vi "Create Group.vi"(4 "Channel Resources (Unset)":string[](array[string]), 5 "Raw Values (F)":bool, 6 "Channel Names":string[](array[string]), 7 "Group Type":refnum<class "GroupAbstract.lvclass">, 8 "error in (no error)":errorcluster, 9 "Publish Config (None)":T1, 10 "Group Info":T2, 11 "TelemetryAPI in":refnum<class "TelemetryAPI.lvclass">) -> (0 "error out":errorcluster, 2 "Group":refnum<class "GroupAbstract.lvclass">, 3 "TelemetryAPI out":refnum<class "TelemetryAPI.lvclass">)   [LabVIEW 2020, in "Volatus.lvlib" / "TelemetryAPI.lvclass"]
uses:
  TelemetryAPI.lvclass
  lv-vecto/Vecto/Group Info.ctl
  lv-vecto/Vecto/Publish Config.ctl
  lv-vecto/Vecto/GroupAbstract/GroupAbstract.lvclass
  TelemetryAPI.lvclass/TelemetryAPI.ctl
  lv-vecto/Vecto/Channel Init.ctl
  lv-vecto/Vecto/ChannelService/Create Group Abstract.vi
  lv-vecto/Vecto/ChannelService/ChannelService.lvclass
  lv-vecto/Vecto/Group Config/Group Config.lvclass
  lv-vecto/Vecto/Vecto.lvlib
  lv-vecto/Vecto/RemoteDataService/RemoteDataService.lvclass
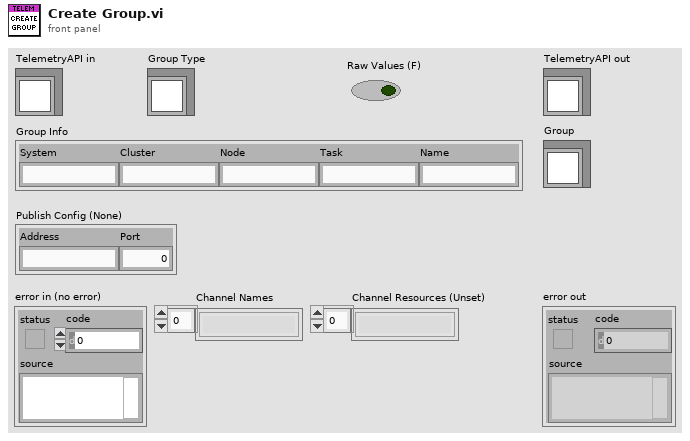
[diagram p1: front panel]
types:
  T1 = typedef "Vecto.lvlib/Publish Config.ctl" = cluster{"Address":string, "Port":u16}
  T2 = typedef "Vecto.lvlib/Group Info.ctl" = cluster{"System":string, "Cluster":string, "Node":string, "Task":string, "Name":string}
  T3 = typedef "Vecto.lvlib/Channel Init.ctl" = cluster{"Name":string, "Resource":string}
  T4 = typedef "Vecto.lvlib/Group Data Type.ctl" = enum16{"Double", "String"}
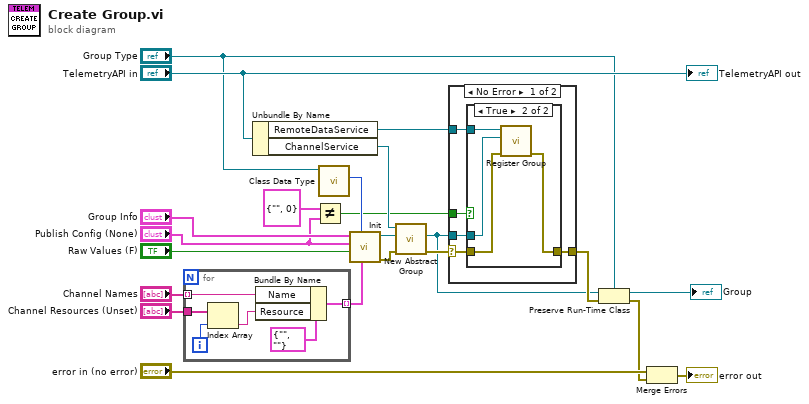
[diagram p0: block diagram]
diagram:
  n1 = for {
    tunnel: "Channel Names" -> [w24] mode=indexing
    tunnel: "Channel Resources (Unset)" -> [w27]
    tunnel: [w23] -> w13 mode=indexing
    i -> [w26]
    n2 = Index Array(array=w27, index=w26) -> (element=w25:string)
    n3 = Bundle By Name(cluster=T3 {"Name"="", "Resource"=""} ("Channel Init"), "Name"=w24, "Resource"=w25) -> (w23:T3)
  }
  n4 = Unbundle By Name("TelemetryAPI in") -> ("RemoteDataService"=w7:refnum<class "RemoteDataService.lvclass">, "ChannelService"=w19:refnum<class "ChannelService.lvclass">)
  n5 = Not Equal?(x=T1 {"Address"="", "Port"=0}, y="Publish Config (None)") -> (x != y?=w6:bool)
  n6 = call "Class Data Type.vi"("GroupAbstract in"="Group Type") -> ("Class Data Type"=w16:T4)  [unwired: 8 in, 2 out]
  n7 = call "Init.vi"("Channels"=w13, "Group Data Type"=w16, "Raw Values (T)"="Raw Values (F)", "Publish Config (None)"="Publish Config (None)", "Group Info"="Group Info") -> ("error out"=w8:errorcluster, "Group Config out"=w12:refnum<class "Group Config.lvclass">)  [unwired: 5 in]
  n8 = call "New Abstract Group.vi"("error in (no error)"=w8, "Group Config"=w12, "ChannelService in"=w19) -> ("error out"=w9:errorcluster, "Group"=w5:refnum<class "GroupAbstract.lvclass">)  [unwired: 6 in, 1 out]
  n9 = case shown="No Error" w9 {
    selector: w9 -> [w30 w39]
    tunnel: w5 -> [w31 _]
    tunnel: w7 -> [w32 _]
    tunnel: w6 -> [w33 _]
    tunnel: [w29 w39] -> w22
    frame No Error {
      n10 = case shown="True" w33 {
        tunnel: w32 -> [_ w38]
        tunnel: w31 -> [_ w37]
        tunnel: w30 -> [w34 w36]
        tunnel: [w34 w35] -> w29
        frame False {
        }
        frame True {
          n11 = call "Register Group.vi"("error in (no error)"=w36, "Group"=w37, "RemoteDataService in"=w38) -> ("error out"=w35:errorcluster)  [unwired: 7 in, 1 out]
        }
      }
    }
    frame Error {
    }
  }
  n12 = Preserve Run-Time Class(object in=w5, error in=w22, 2:"Group Type") -> (object out=→"Group":refnum<class "GroupAbstract.lvclass">, error out=w1:errorcluster)
  n13 = Merge Errors("error in (no error)", w1) -> (→"error out":errorcluster)
  "TelemetryAPI out" <- "TelemetryAPI in"
